vi "Moving Average.vi"(11 "Numeric in":dbl) -> (3 "Numeric out":dbl)   [LabVIEW 2012]
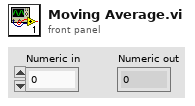
[diagram p1: front panel]
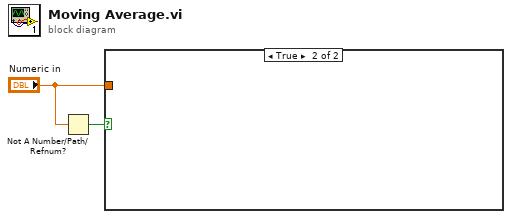
[diagram p0: block diagram]
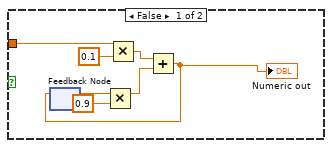
[diagram p2: hidden frame]
diagram:
  n1 = Not A Number/Path/Refnum?(number/path/refnum="Numeric in") -> (NaN/Path/Refnum?=w2:bool)
  n2 = case shown="True" w2 {
    tunnel: "Numeric in" -> [w6 _]
    frame False {
      n3 = feedback #1() -> (w9:dbl)  [unwired: 1 in]
      n4 = Multiply(x=w9, y=0.9) -> (x*y=w5:dbl)
      n5 = Multiply(x=w6, y=0.1) -> (x*y=w8:dbl)
      n6 = Add(x=w8, y=w5) -> (x+y=w3:dbl)
      "Numeric out" <- w3
      n7 = feedback-in #1(w3) -> ()
    }
    frame True {
    }
  }
